vi "Result.vi"(8 "error in (no error)":errorcluster, 10 "Result":T1={"Name"="", "Message"="", "Description"="", "Status"=enum."Passed", "Result Type"=enum."Case", "Execution Time"=0.0}, 11 "Execution UI In":refnum<class "Execution UI.lvclass">) -> (0 "error out":errorcluster)   [LabVIEW 2020, in "Execution UI.lvclass"]
uses:
  Execution UI.lvclass
  C:/Git/astemes-lunit/source/Application Framework/Process Classes/Process/Process.lvclass
  Core/Result/Result.ctl
  Core/Result/Status.ctl
  Core/Result/Type.ctl
  Application Framework/Process Classes/Process/Process.lvclass/Process.ctl
  Application Framework/Process Classes/Process/Process.lvclass
  Core/Result/Result.lvlib
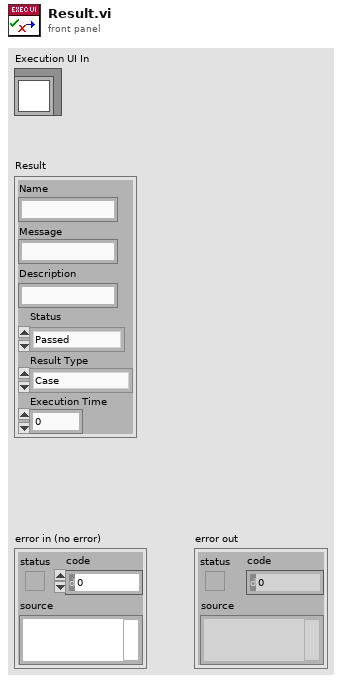
[diagram p1: front panel]
types:
  T1 = typedef "Result.lvlib/Result.ctl" = cluster{"Name":string, "Message":string, "Description":string, "Status":T2, "Result Type":T3, "Execution Time":dbl}
  T2 = typedef "Result.lvlib/Status.ctl" = enum16{"", "Passed", "Failed", "Error", "Skipped", "Setup Error", "Broken", "Teardown Error"}
  T3 = typedef "Result.lvlib/Type.ctl" = enum16{"Method", "Case", "Suite", "Pass", "Fail", "Skip", "Pass if", "Fail if", "Pass if Error", "Fail if Error", "Pass if Equal", "Fail if Equal"}
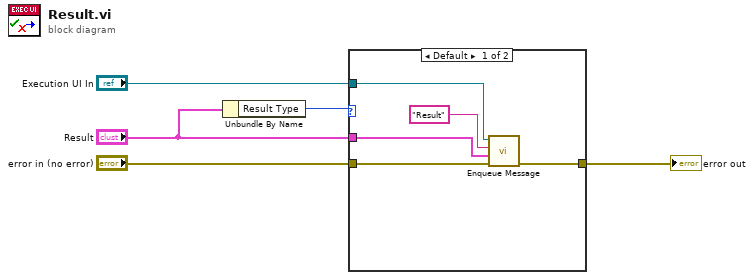
[diagram p0: block diagram]
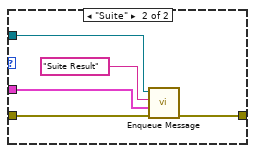
[diagram p2: hidden frame]
diagram:
  n1 = Unbundle By Name("Result") -> ("Result Type"=w1:T3)
  n2 = case shown="Default" w1 {
    tunnel: "Execution UI In" -> [w10 w15]
    tunnel: "error in (no error)" -> [w8 w13]
    tunnel: "Result" -> [w7 w12]
    tunnel: [w6 w11] -> w2
    frame Default {
      n3 = call "Enqueue Message.vi"("error in (no error)"=w8, "Message Data"=w7, "Message"="Result", "Process In"=w10) -> ("error out"=w6:errorcluster)  [unwired: 6 in, 1 out]
    }
    frame "Suite" {
      n4 = call "Enqueue Message.vi"("error in (no error)"=w13, "Message Data"=w12, "Message"="Suite Result", "Process In"=w15) -> ("error out"=w11:errorcluster)  [unwired: 6 in, 1 out]
    }
  }
  "error out" <- w2
